vi "Check Persistent Core Actor.vi"(10 "Persistent Core Actor":refnum<class "Actor.lvclass">) -> (2 "Error":errorcluster)   [LabVIEW 2025, in "jettl.lvlib"]
uses:
  jettl.lvlib
  Actor/Actor.lvclass
  Error/Error.lvlib
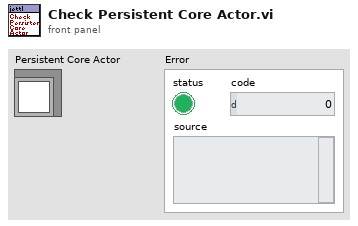
[diagram p1: front panel]
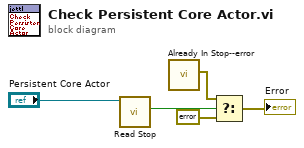
[diagram p0: block diagram]
diagram:
  n1 = call-dynamic "Read Stop.vi"("Actor in"="Persistent Core Actor") -> ("Stop"=w3:bool)  [unwired: 10 in]
  n2 = call "Already In Stop--error.vi"() -> ("Error"=w4:errorcluster)  [unwired: 11 in]
  n3 = Select(t=w4, s=w3, f=errorcluster {"status"=FALSE, "code"=0, "source"=""}) -> (s? t:f=→"Error":errorcluster)
